vi "ENPH 354 Assignment 1 - Q4.vi"() -> ()   [LabVIEW 2021]
panel:
  out "String":string
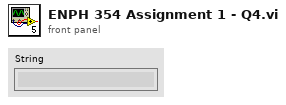
[diagram p1: front panel]
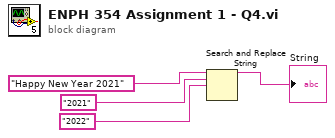
[diagram p0: block diagram]
diagram:
  n1 = Search and Replace String(input string="Happy New Year 2021", search string="2021", replace string="2022") -> (result string=→"String":string)  [unwired: 5 in, 3 out]
